vi "test_variance_map.vi"() -> ()   [LabVIEW 2009]
doc: "Copyright (C) 2009, Stepan A. Baranov\nweb: http://www.OCTLab.org/\nemail: stepan@baranov.su"
uses:
  OCTLib.dll
  <vilib>/Analysis/NI_AALBase.lvlib
panel:
  out "version":string
  out "name":string
  out "error out":errorcluster
  out "cell height":i32
  out "cell width":i32
  out "A-scan size":i32
  out "# of A-scans":i32
  in  "Small/Big":bool
  out "loop #":i32
  out "RSM_STAT time":u32
  out "LabView time":u32
  out "RSM_STAT Array":dbl[][](array[numeric])
  out "LabView Array":dbl[][](array[numeric])
  in  "stop":bool
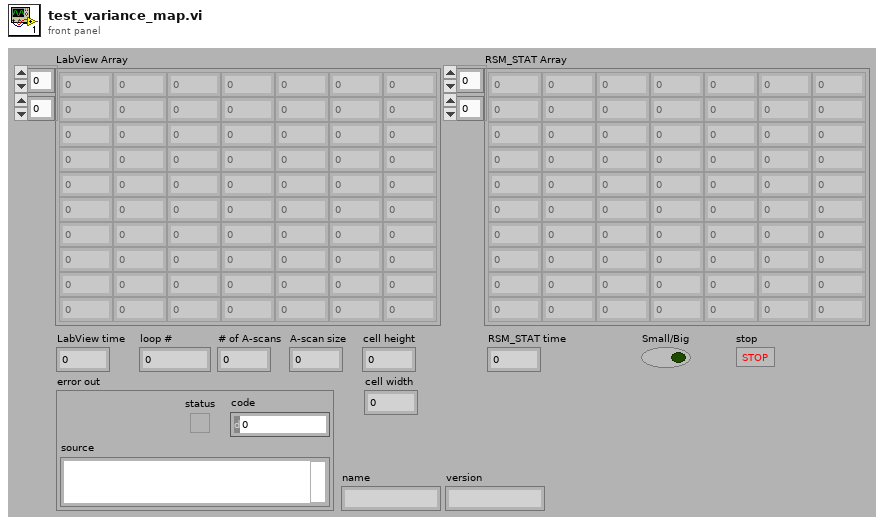
[diagram p1: front panel]
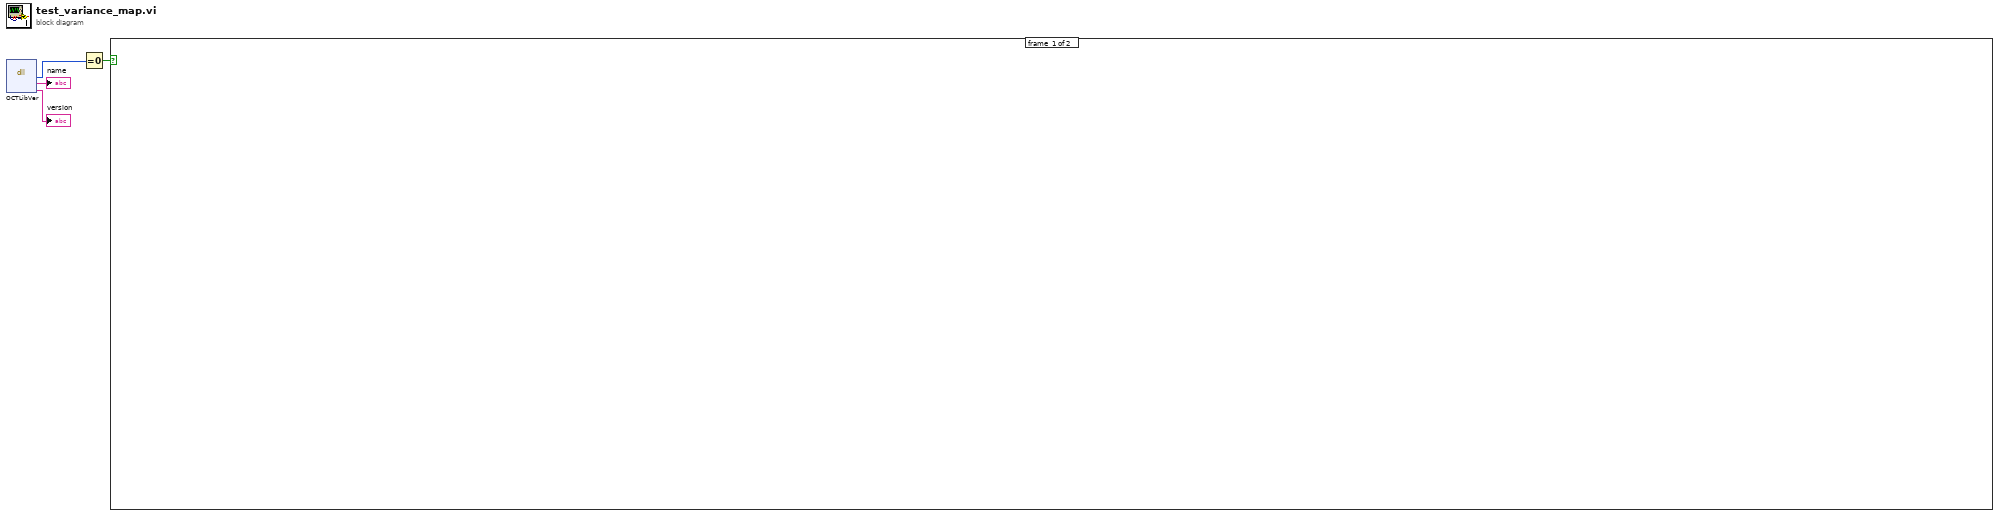
[diagram p0: block diagram]
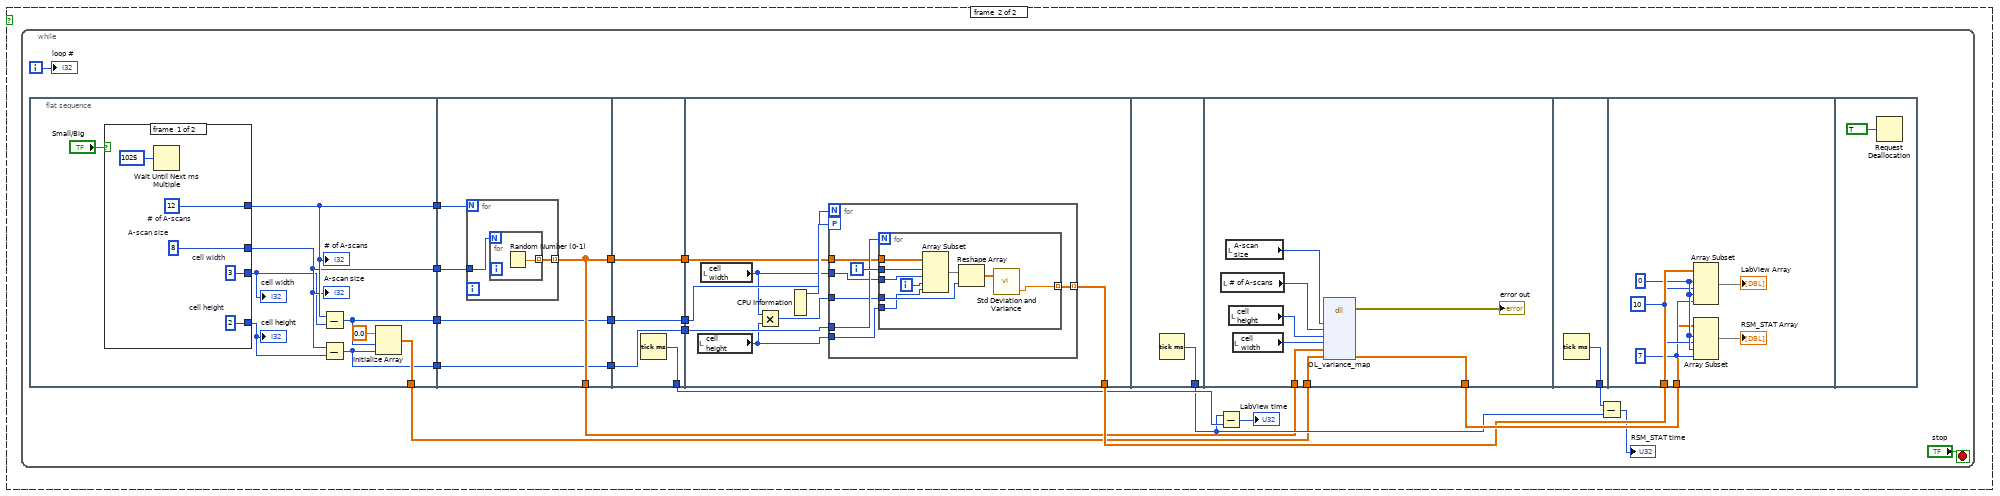
[diagram p2: hidden frame]
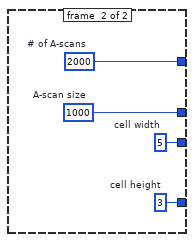
[diagram p3: hidden frame]
diagram:
  n1 = dll-call lib="OCTLib.dll" fn="OCTLibVer"() -> ("status"=w4:i8, "name"=→"name":string, "version"=→"version":string)  [unwired: 5 in, 2 out]
  n2 = Equal To 0?(x=w4) -> (x = 0?=w3:bool)
  n3 = case shown="True" w3 {
    frame #0 {
    }
    frame #1 {
      n4 = while {
        i -> [w17]
        stop <- "stop" stop-if-true
        n5 = flat-sequence {
          tunnel: [w31] -> w13
          tunnel: [w33] -> w12
          tunnel: [w30] -> w11
          tunnel: [w27] -> w6
          tunnel: [w26] -> w5
          tunnel: [w48] -> w16
          tunnel: [w48] -> w14
          tunnel: w13 -> [w47]
          tunnel: w12 -> [w46]
          tunnel: [w44] -> w10
          tunnel: [w45] -> w8
          tunnel: w6 -> [w45]
          tunnel: w5 -> [w44]
          tunnel: [w55] -> w22
          tunnel: [w54] -> w15
          tunnel: w14 -> [w54]
          tunnel: w10 -> [w53]
          tunnel: [w53] -> w9
          tunnel: w8 -> [w52]
          tunnel: [w52] -> w7
          tunnel: [w62] -> w23
          tunnel: w15 -> [w56]
          tunnel: w9 -> [w61]
          tunnel: w7 -> [w60]
          tunnel: [w80] -> w19
          tunnel: w16 -> [w85]
          tunnel: [w88] -> w24
          tunnel: w11 -> [w82]
          tunnel: [w89] -> w20
          tunnel: w24 -> [w90]
          tunnel: w23 -> [w96]
          frame #0 {
            n6 = case shown="False" "Small/Big" {
              tunnel: [w38 w42] -> w33
              tunnel: [w39 w43] -> w31
              tunnel: [w36 w41] -> w28
              tunnel: [w35 w40] -> w29
              frame #0 {
                w35 = 2  # cell height
                w36 = 3  # cell width
                w39 = 8  # A-scan size
                w38 = 12  # # of A-scans
                n7 = Wait Until Next ms Multiple(millisecond multiple=u32 1025) -> ()  [unwired: 1 out]
              }
              frame #1 {
                w40 = 3  # cell height
                w41 = 5  # cell width
                w43 = 1000  # A-scan size
                w42 = 2000  # # of A-scans
              }
            }
            "# of A-scans" <- w33
            "A-scan size" <- w31
            "cell width" <- w28
            "cell height" <- w29
            n8 = Subtract(x=w33, y=w28) -> (x-y=w27:i32)
            n9 = Subtract(x=w31, y=w29) -> (x-y=w26:i32)
            n10 = Initialize Array(0.0 ("element"), w27, w26) -> (w30:dbl[][])
          }
          frame #1 {
            n11 = for {
              N: w46 -> [_]
              tunnel: w47 -> [w50]
              tunnel: [w49] -> w48 mode=indexing
              n12 = for {
                N: w50 -> [_]
                tunnel: [w51] -> w49 mode=indexing
                n13 = Random Number (0-1)() -> (number: 0 to 1=w51:dbl)
              }
            }
          }
          frame #2 {
            n14 = Tick Count (ms)() -> (millisecond timer value=w55:u32)
          }
          frame #3 {
            n15 = local read "cell height"() -> (w57:i32)
            n16 = local read "cell width"() -> (w58:i32)
            n17 = Multiply(x=w58, y=w57) -> (x*y=w59:i32)
            n18 = CPU Information() -> (4:w63:i32)  [unwired: 3 out]
            n19 = for {
              N: w60 -> [_]
              tunnel: [w69] -> w62 mode=indexing
              workers-P: w63 -> [_]
              tunnel: w61 -> [w68]
              tunnel: w59 -> [w67]
              tunnel: w58 -> [w66]
              tunnel: w57 -> [w65]
              tunnel: w56 -> [w64]
              i -> [w70]
              n20 = for {
                N: w68 -> [_]
                tunnel: w70 -> [w79]
                tunnel: [w71] -> w69 mode=indexing
                tunnel: w67 -> [w76]
                tunnel: w66 -> [w75]
                tunnel: w65 -> [w74]
                tunnel: w64 -> [w73]
                i -> [w78]
                n21 = Array Subset(array=w73, index (row)=w79, length (row)=w75, index (col)=w78, length (col)=w74) -> (w77:dbl[][])
                n22 = Reshape Array(w77, w76) -> (w72:dbl[])
                n23 = call <vilib>:"Std Deviation and Variance.vi"("X"=w72) -> ("variance"=w71:dbl)  [unwired: 1 in, 2 out]
              }
            }
          }
          frame #4 {
            n24 = Tick Count (ms)() -> (millisecond timer value=w80:u32)
          }
          frame #5 {
            n25 = local read "# of A-scans"() -> (w86:i32)
            n26 = local read "A-scan size"() -> (w87:i32)
            n27 = local read "cell height"() -> (w84:i32)
            n28 = local read "cell width"() -> (w83:i32)
            n29 = dll-call lib="OCTLib.dll" fn="OL_variance_map"("A-scan size"=w87, "# of A-scan"=w86, "cell height"=w84, "cell width"=w83, "input"=w85, "data"=w82) -> (error out=→"error out":errorcluster, "data"=w88:dbl[][])  [unwired: 9 in, 1 out]
          }
          frame #6 {
            n30 = Tick Count (ms)() -> (millisecond timer value=w89:u32)
          }
          frame #7 {
            w93 = 10 ("length")
            w92 = 7 ("length")
            w94 = 0 ("index")
            n31 = Array Subset(array=w96, index (row)=w94, length (row)=w93, index (col)=w94, length (col)=w92) -> (→"LabView Array":dbl[][])
            n32 = Array Subset(array=w90, index (row)=w94, length (row)=w93, index (col)=w94, length (col)=w92) -> (→"RSM_STAT Array":dbl[][])
          }
          frame #8 {
            n33 = Request Deallocation(TRUE ("flag")) -> ()
          }
        }
        n34 = Subtract(x=w19, y=w22) -> (x-y=→"LabView time":u32)
        n35 = Subtract(x=w20, y=w19) -> (x-y=→"RSM_STAT time":u32)
        "loop #" <- w17
      }
    }
  }
